vi "SetElement.vi"(9 "Destination":T4={"Subsystem Id"=90, "Node Id"=1, "Component Id"=1}, 10 "RequestIDRec":T1, 11 "Source":T4={"Subsystem Id"=3, "Node Id"=1, "Component Id"=1}) -> (2 "Encoded JAUS Message":string)   [LabVIEW 2009]
uses:
  Support Files/Address.ctl
  Support Files/RequestIDRec.ctl
  Support Files/ElementRec.ctl
  Support Files/LocalWaypointRec.ctl
panel:
  out "payload":string
  in  "Command Code":string="\u0004\u001a"
  # "According to the FAQ, this is supposed to be serialized waypoint message\nhttp://usaric.org/simplemachinesforum/index.php?PHPSESSID=9faba26d82c8900d007d94b652b30214&topic=32.msg103#msg103"
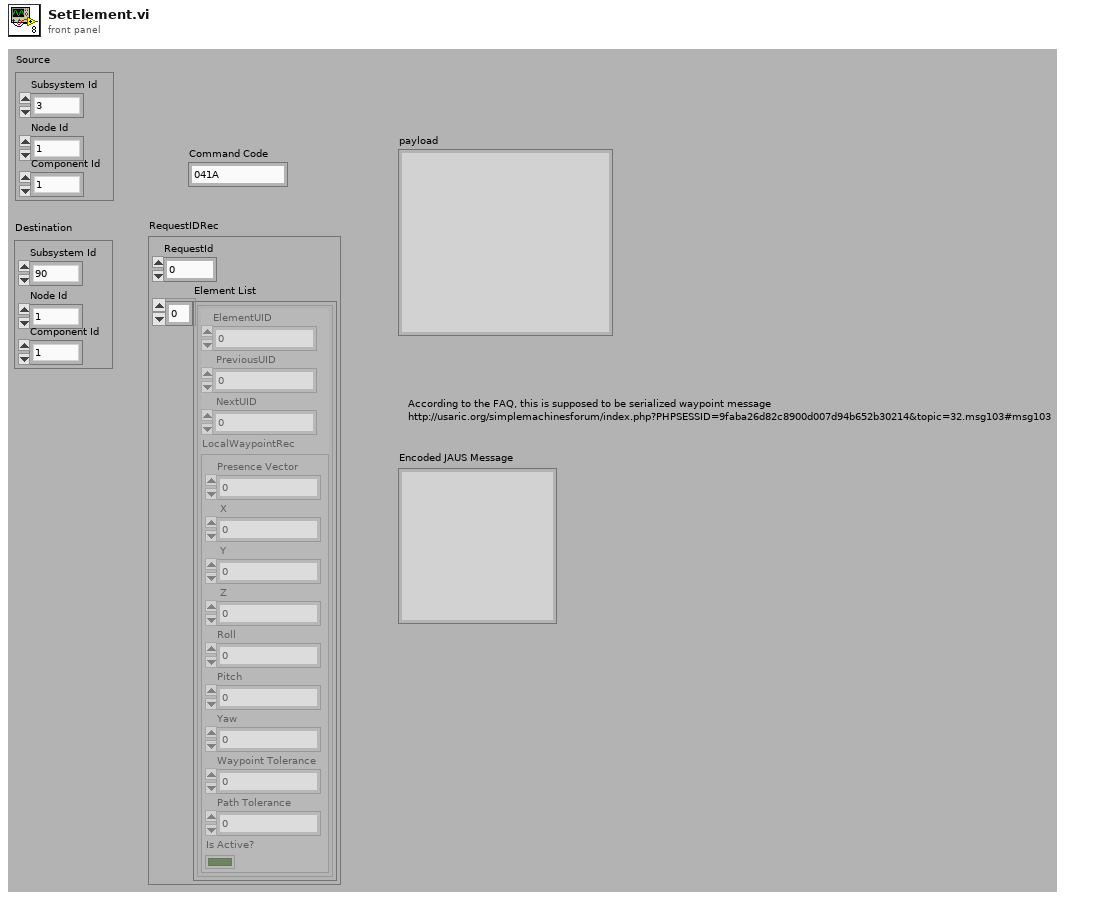
[diagram p1: front panel]
types:
  T1 = typedef "RequestIDRec.ctl" = cluster{"RequestId":u8, "Element List":T2[]}
  T2 = typedef "ElementRec.ctl" = cluster{"ElementUID":u16, " PreviousUID":u16, " NextUID":u16, "LocalWaypointRec":T3}
  T3 = typedef "LocalWaypointRec.ctl" = cluster{"Presence Vector":u8, " X":dbl, " Y":dbl, " Z":dbl, "Roll":dbl, "Pitch":dbl, "Yaw":dbl, "Waypoint Tolerance":dbl, "Path Tolerance":dbl, "Is Active?":bool}
  T4 = typedef "Address.ctl" = cluster{"Subsystem Id":u16, "Node Id":u8, "Component Id":u8}
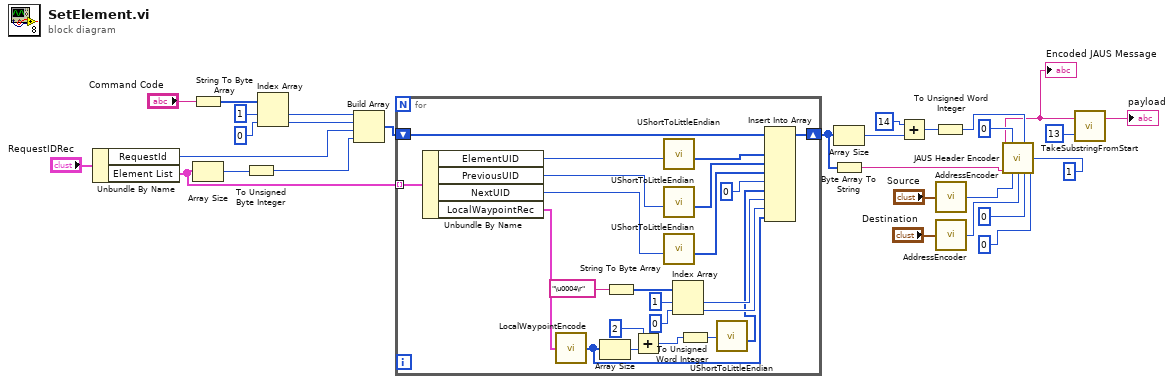
[diagram p0: block diagram]
diagram:
  n1 = Unbundle By Name("RequestIDRec") -> ("RequestId"=w9:u8, "Element List"=w6:T2[])
  n2 = String To Byte Array(string="Command Code") -> (unsigned byte array=w15:u8[])
  n3 = Array Size(array=w6) -> (size(s)=w5:i32)
  n4 = To Unsigned Byte Integer(number=w5) -> (unsigned 8bit integer=w4:u8)
  n5 = Index Array(array=w15, index #1=1 ("index"), index #2=0 ("index")) -> (element #1=w12:u8, element #2=w11:u8)
  n6 = Build Array(w12, w11, w9, w4) -> (w8:u8[])
  n7 = for {
    tunnel: w6 -> [w52] mode=indexing
    shift-right: [w49] -> w7
    shift-left: w8 -> [w51]
    n8 = Unbundle By Name(w52) -> ("ElementUID"=w48:u16, "PreviousUID"=w46:u16, "NextUID"=w44:u16, "LocalWaypointRec"=w50:T3)
    n9 = call "LocalWaypointEncode.vi"("LocalWaypointRec"=w50) -> ("Array"=w37:u8[])
    n10 = Array Size(array=w37) -> (size(s)=w42:i32)
    n11 = String To Byte Array(string="\u0004\r") -> (unsigned byte array=w41:u8[])
    n12 = Add(x=2, y=w42) -> (x+y=w32:i32)
    n13 = call "UShortToLittleEndian.vi"("Number"=w48) -> ("byte array"=w47:u8[])  [unwired: 10 in]
    n14 = call "UShortToLittleEndian.vi"("Number"=w46) -> ("byte array"=w45:u8[])  [unwired: 10 in]
    n15 = call "UShortToLittleEndian.vi"("Number"=w44) -> ("byte array"=w43:u8[])  [unwired: 10 in]
    n16 = Index Array(array=w41, index #1=1 ("index"), index #2=0 ("index")) -> (element #1=w35:u8, element #2=w34:u8)
    n17 = To Unsigned Word Integer(number=w32) -> (unsigned 16bit integer=w31:u16)
    n18 = call "UShortToLittleEndian.vi"("Number"=w31) -> ("byte array"=w30:u8[])  [unwired: 10 in]
    n19 = Insert Into Array(array=w51, new element #1=w47, new element #2=w45, new element #3=w43, new element #4=u8 0 ("new element/subarray"), new element #5=w30, new element #6=w35, new element #7=w34, new element #8=w37) -> (w49:u8[])  [unwired: 1 in]
  }
  n20 = Array Size(array=w7) -> (size(s)=w20:i32)
  n21 = Byte Array To String(unsigned byte array=w7) -> (string=w23:string)
  n22 = Add(x=14, y=w20) -> (x+y=w19:i32)
  n23 = To Unsigned Word Integer(number=w19) -> (unsigned 16bit integer=w16:u16)
  n24 = call "AddressEncoder.vi"("Address Cluster"="Source") -> ("Address"=w29:u32)
  n25 = call "AddressEncoder.vi"("Address Cluster"="Destination") -> ("Address"=w28:u32)
  n26 = call "JAUS Header Encoder.vi"("Message Type (0-5)"=u8 0, "Data Size (8-23)"=w16, "Priority(40-41)"=u8 1, "Payload"=w23, "Source ID (80-95)"=w29, "Destination ID (48-79)"=w28, "Data Flags (46-47)"=u8 0, "Ack/Nak (44-45)"=u8 0) -> ("Encoded JAUS Message"=w3:string)  [unwired: 7 in]
  "Encoded JAUS Message" <- w3
  n27 = call "TakeSubstringFromStart.vi"("offset"=13, "string"=w3) -> ("string after offset"=→"payload":string)  [unwired: 1 out]
